vi "Init System.vi"(8 "error in (no error)":errorcluster, 11 "Application Name":string) -> (0 "error out":errorcluster)   [LabVIEW 2016, in "System.lvlib"]
uses:
  System.lvlib
  Controls/Control_Data Functions.ctl
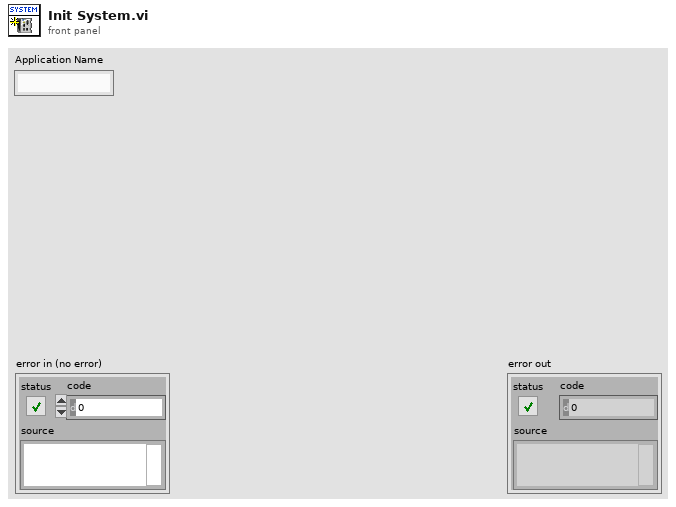
[diagram p1: front panel]
types:
  T1 = typedef "System.lvlib/Control_Data Functions.ctl" = enum16{"Get", "Set", "Release"}
  T2 = typedef "System.lvlib/Control_Variant Data Reference.ctl" = refnum<data-value>
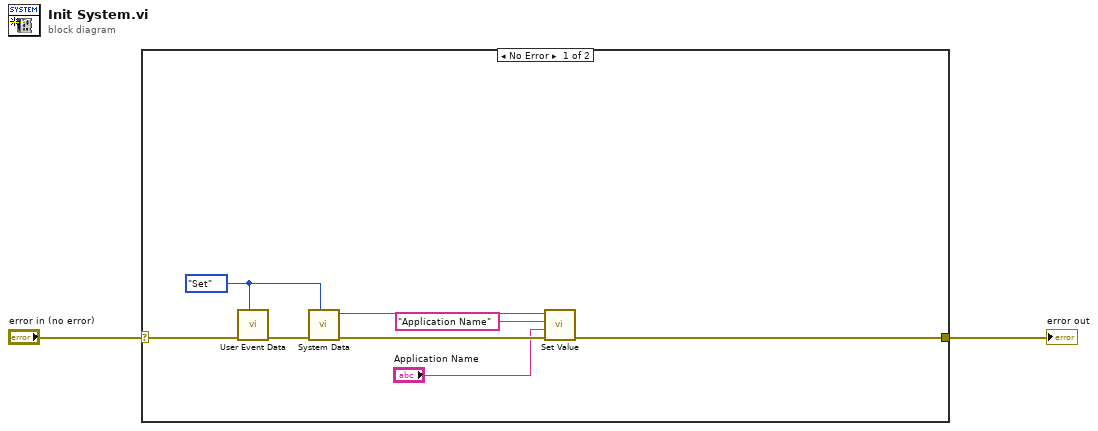
[diagram p0: block diagram]
diagram:
  n1 = case shown="No Error" "error in (no error)" {
    selector: "error in (no error)" -> [w10 w11]
    tunnel: [w6 w11] -> w1
    frame No Error {
      w8 = Control_Data_Functions."Set" ("Data Functions")
      n2 = call "User Event Data.vi"("Data Functions"=w8, "error in (no error)"=w10) -> ("error out"=w9:errorcluster)  [unwired: 8 in, 1 out]
      n3 = call "System Data.vi"("Data Functions"=w8, "error in (no error)"=w9) -> ("error out"=w7:errorcluster, "System Data Reference"=w5:T2)  [unwired: 8 in]
      n4 = call "Set Value.vi"("error in (no error)"=w7, "Value"="Application Name", "Name"="Application Name", "Data Reference"=w5) -> ("error out"=w6:errorcluster)  [unwired: 7 in]
    }
    frame Error {
    }
  }
  "error out" <- w1
